vi "Insight_Read_Laser_Parameters_from_File.vi"(8 "error in (no error)":errorcluster, 10 "Actual Laser Settings":T2={"Clock Rate (MHz)"=400.0, "Sample Pts"=0, "Total Sweep Pts"=0, "Total Pts Increment"=4, "Reversal Index"=0, "Sweep Efficiency (%)"=nan, "Duty Cycle (%)"=nan, "Repetition Rate (kHz)"=nan, "Sweep Rate (kHz)"=nan, "Min Wavelength (nm)"=nan, "Max Wavelength (nm)"=nan, "Power (mW)"=nan, "Power Profile"=enum."FLAT", "Edge Roll-off (dB)"=0.0, "Sample Clock Delay (nsec)"=0.0, "Sweep Start Delay (nsec)"=0.0, "Data Valid Delay (nsec)"=0.0, "Optical Freq. Step (GHz)"=0.1, "Sweep Start Trigger Edge"=enum."BOTH", "WL Sweep Direction?"=enum."Increase"} {"Sweep Rate (kHz)" format="%#.2g"; "Sweep Efficiency (%)" format="%#.3g"; "Repetition Rate (kHz)" format="%#.2g"}, 11 "Save Data Path in":path) -> (0 "error out":errorcluster, 1 "Data Valid Vector":u32[](array[numeric]), 2 "Actual Laser Settings Out":T2={"Clock Rate (MHz)"=400.0, "Sample Pts"=0, "Total Sweep Pts"=0, "Total Pts Increment"=4, "Reversal Index"=0, "Sweep Efficiency (%)"=nan, "Duty Cycle (%)"=nan, "Repetition Rate (kHz)"=nan, "Sweep Rate (kHz)"=nan, "Min Wavelength (nm)"=nan, "Max Wavelength (nm)"=nan, "Power (mW)"=nan, "Power Profile"=enum."FLAT", "Edge Roll-off (dB)"=0.0, "Sample Clock Delay (nsec)"=0.0, "Sweep Start Delay (nsec)"=0.0, "Data Valid Delay (nsec)"=0.0, "Optical Freq. Step (GHz)"=0.1, "Sweep Start Trigger Edge"=enum."BOTH", "WL Sweep Direction?"=enum."Increase"} {"Sweep Rate (kHz)" format="%#.2g"; "Sweep Efficiency (%)" format="%#.3g"; "Repetition Rate (kHz)" format="%#.2g"}, 3 "Hold Data Vector":u32[](array[numeric]))   [LabVIEW 2011]
doc: "Insight Photonic Solutions\n\nThis VI reads laser parameters, the Data Valid Vector and the Hold Data Vector (aka Invalid Points) from three text files, \"Laser Parameters.txt\", \"DVV.txt\" and \"Hold Data Vector.txt\". Use this VI to pass information from the laser standalone program into your data acquisition program.\n\nver 1.0 - original release\nver 1.1 - updated the order of parameters, added Sweep Efficiency (%)\nver 1.2 - read Hold Data Vector and ouput integer array. \nver 3.5 - updated to use new Actual Laser Settings cluster with Sweep Rate, Total Points Increment, Reversal Index, Edge Roll-off of Gaussian Profile, Min Wavelength (formerly Beginning Wavelength) and Max Wavelength (formerly Ending Wavelength)"
uses:
  Start_Sweep_Trigger.ctl
  <vilib>/Utility/file.llb/Read From Spreadsheet File (I64).vi
  <vilib>/Utility/file.llb/Read From Spreadsheet File (string).vi
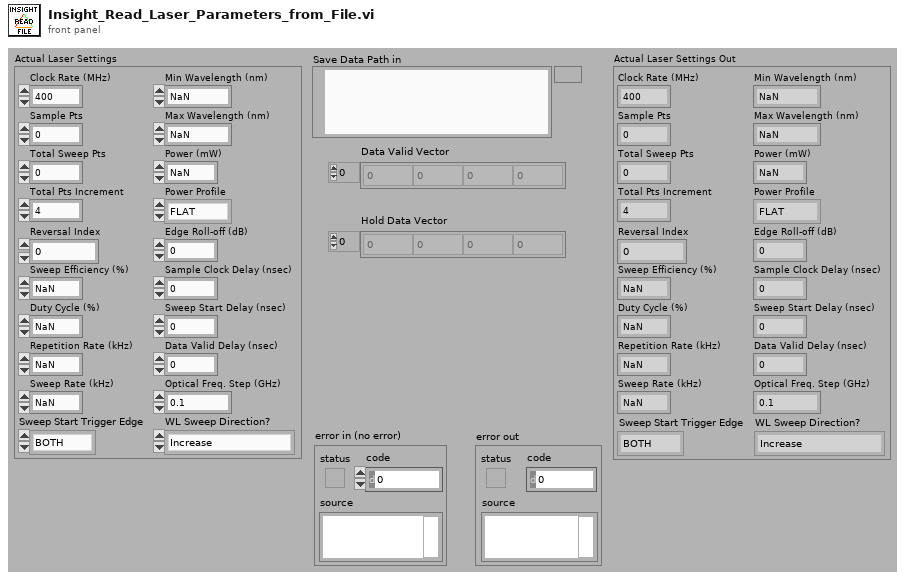
[diagram p1: front panel]
types:
  T1 = typedef "Start_Sweep_Trigger.ctl" = enum16{"RISing", "FALLing", "BOTH"}
  T2 = cluster{"Clock Rate (MHz)":dbl, "Sample Pts":u32, "Total Sweep Pts":i32, "Total Pts Increment":u32, "Reversal Index":u32, "Sweep Efficiency (%)":dbl, "Duty Cycle (%)":dbl, "Repetition Rate (kHz)":dbl, "Sweep Rate (kHz)":dbl, "Min Wavelength (nm)":dbl, "Max Wavelength (nm)":dbl, "Power (mW)":dbl, "Power Profile":enum16{"FLAT", "GAUSsian"}, "Edge Roll-off (dB)":dbl, "Sample Clock Delay (nsec)":dbl, "Sweep Start Delay (nsec)":dbl, "Data Valid Delay (nsec)":dbl, "Optical Freq. Step (GHz)":dbl, "Sweep Start Trigger Edge":T1, "WL Sweep Direction?":enum16{"Increase", "Decrease", "Bidirectional_Increase", "Bidirectional_Decrease"}}
  T3 = enum16{"Increase", "Decrease", "Bidirectional_Increase", "Bidirectional_Decrease"}
  T4 = cluster{"[0]":dbl, "[1]":dbl, "[2]":dbl, "[3]":dbl, "[4]":dbl, "[5]":dbl, "[6]":dbl, "[7]":dbl, "[8]":dbl, "[9]":dbl, "[10]":dbl, "[11]":dbl}
  T5 = cluster{"[0]":dbl, "[1]":dbl, "[2]":dbl, "[3]":dbl, "[4]":dbl}
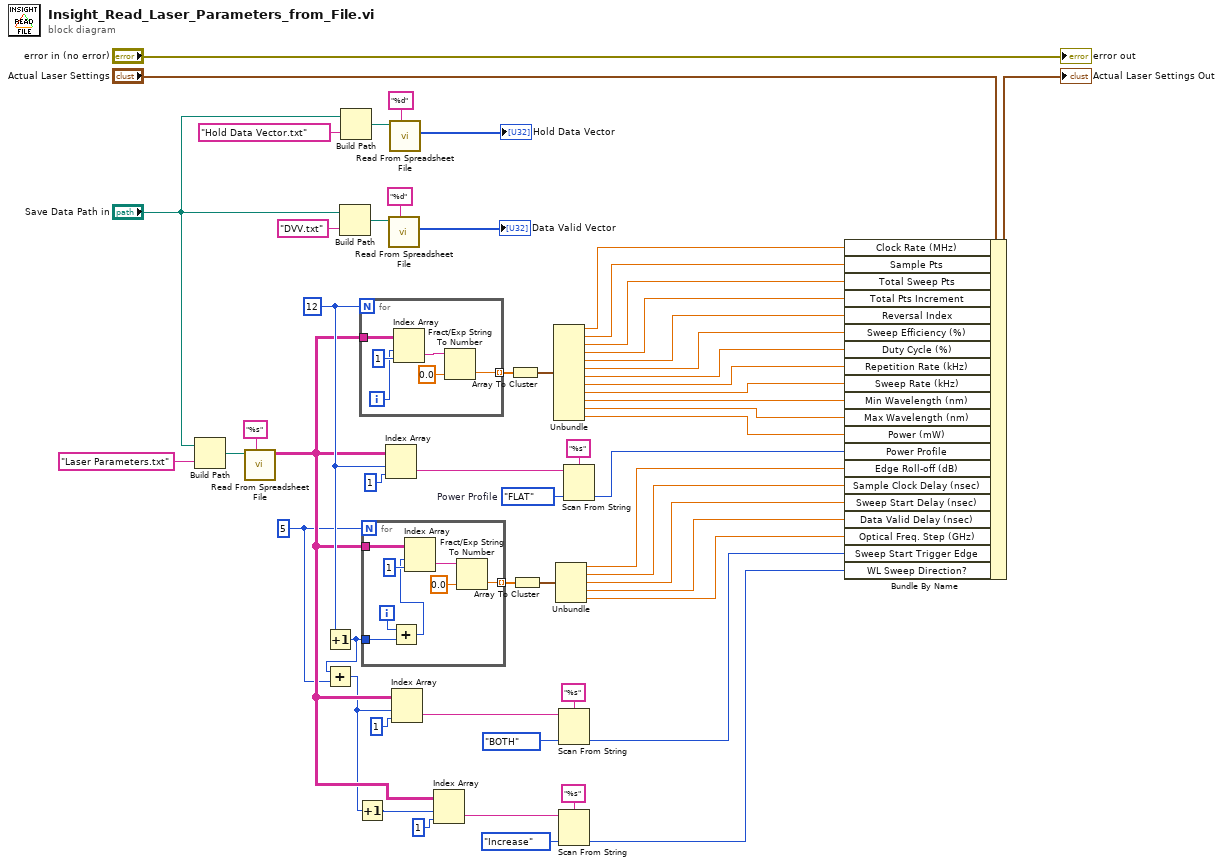
[diagram p0: block diagram]
diagram:
  w2 = 5
  w48 = enum16{"FLAT", "GAUSsian"}."FLAT"  # Power Profile
  w20 = 12
  n1 = Build Path(base path="Save Data Path in", name or relative path="Laser Parameters.txt" ("time format string (%c)")) -> (appended path=w51:path)
  n2 = call-poly <vilib>:"Read From Spreadsheet File.vi"("format (%s)"="%s" ("format (%.3f)"), "file path (dialog if empty)"=w51) -> ("all rows"=w8:string[][])  [unwired: 5 in, 4 out]
  n3 = Increment(x=w20) -> (x+1=w3:i32)
  n4 = Add(x=w3, y=w2) -> (x+y=w1:i32)
  n5 = Build Path(base path="Save Data Path in", name or relative path="DVV.txt" ("time format string (%c)")) -> (appended path=w55:path)
  n6 = Build Path(base path="Save Data Path in", name or relative path="Hold Data Vector.txt" ("time format string (%c)")) -> (appended path=w35:path)
  n7 = Increment(x=w1) -> (x+1=w7:i32)
  n8 = for {
    N: w20 -> [_]
    tunnel: w8 -> [w60]
    tunnel: [w59] -> w50 mode=indexing
    i -> [w58]
    n9 = Index Array(array=w60, index (row)=w58, index (col)=1) -> (element=w63:string)
    n10 = Fract/Exp String To Number(string=w63, default (0 dbl)=0.0 ("default (0 DBL)")) -> (number=w59:dbl)  [unwired: 2 in, 1 out]
  }
  n11 = for {
    N: w2 -> [_]
    tunnel: w8 -> [w68]
    tunnel: [w67] -> w44 mode=indexing
    tunnel: w3 -> [w66]
    i -> [w65]
    n12 = Add(x=w65, y=w66) -> (x+y=w64:i32)
    n13 = Index Array(array=w68, index (row)=w64, index (col)=1) -> (element=w71:string)
    n14 = Fract/Exp String To Number(string=w71, default (0 dbl)=0.0 ("default (0 DBL)")) -> (number=w67:dbl)  [unwired: 2 in, 1 out]
  }
  n15 = Index Array(array=w8, index (row)=w20, index (col)=1 ("disabled index (col)")) -> (element=w46:string)
  n16 = call-poly <vilib>:"Read From Spreadsheet File.vi"("format (%d)"="%d" ("format (%.3f)"), "file path (dialog if empty)"=w55) -> ("first row"=→"Data Valid Vector":i64[])  [unwired: 5 in, 4 out]
  n17 = call-poly <vilib>:"Read From Spreadsheet File.vi"("format (%d)"="%d" ("format (%.3f)"), "file path (dialog if empty)"=w35) -> ("first row"=→"Hold Data Vector":i64[])  [unwired: 5 in, 4 out]
  n18 = Index Array(array=w8, index (row)=w1, index (col)=1 ("disabled index (col)")) -> (element=w15:string)
  n19 = Index Array(array=w8, index (row)=w7, index (col)=1 ("disabled index (col)")) -> (element=w6:string)
  n20 = Array To Cluster(array=w50) -> (cluster=w42:T4)
  n21 = Array To Cluster(array=w44) -> (cluster=w43:T5)
  n22 = Unbundle(w42) -> ("[0]"=w41:dbl, "[1]"=w40:dbl, "[2]"=w39:dbl, "[3]"=w27:dbl, "[4]"=w26:dbl, "[5]"=w28:dbl, "[6]"=w29:dbl, "[7]"=w30:dbl, "[8]"=w16:dbl, "[9]"=w17:dbl, "[10]"=w18:dbl, "[11]"=w19:dbl)
  n23 = Unbundle(w43) -> ("[0]"=w21:dbl, "[1]"=w22:dbl, "[2]"=w23:dbl, "[3]"=w24:dbl, "[4]"=w25:dbl)
  n24 = Scan From String(format string="%s", input string=w15, default 1=Start_Sweep_Trigger."BOTH" ("Sweep Start Trigger Edge")) -> (output 1=w11:T1)  [unwired: 2 in, 3 out]
  n25 = Scan From String(format string="%s", input string=w6, default 1=T3."Increase" ("WL Sweep Direction?")) -> (output 1=w4:T3)  [unwired: 2 in, 3 out]
  n26 = Scan From String(format string="%s", input string=w46, default 1=w48) -> (output 1=w45:enum16{"FLAT", "GAUSsian"})  [unwired: 2 in, 3 out]
  n27 = Bundle By Name(cluster="Actual Laser Settings", "Clock Rate (MHz)"=w41, "Sample Pts"=w40, "Total Sweep Pts"=w39, "Total Pts Increment"=w27, "Reversal Index"=w26, "Sweep Efficiency (%)"=w28, "Duty Cycle (%)"=w29, "Repetition Rate (kHz)"=w30, "Sweep Rate (kHz)"=w16, "Min Wavelength (nm)"=w17, "Max Wavelength (nm)"=w18, "Power (mW)"=w19, "Power Profile"=w45, "Edge Roll-off (dB)"=w21, "Sample Clock Delay (nsec)"=w22, "Sweep Start Delay (nsec)"=w23, "Data Valid Delay (nsec)"=w24, "Optical Freq. Step (GHz)"=w25, "Sweep Start Trigger Edge"=w11, "WL Sweep Direction?"=w4) -> (→"Actual Laser Settings Out":T2)
  "error out" <- "error in (no error)"
